vi "Set Temperature.vi"(8 "error in (no error)":errorcluster, 11 "CCDCamera in":refnum<class "CCDCamera.lvclass">) -> (0 "error out":errorcluster, 3 "CCDCamera out":refnum<class "CCDCamera.lvclass">)   [LabVIEW 2018, in "CCDCamera.lvclass"]
uses:
  CCDCamera.lvclass
  C:/Users/observer/Desktop/SPARC4_ACS/SPARC4_ACS/Simulated_CCD_Camera/Simulated_CCD_Camera.lvclass
  Simulated_CCD_Camera/Simulated_CCD_Camera.lvclass
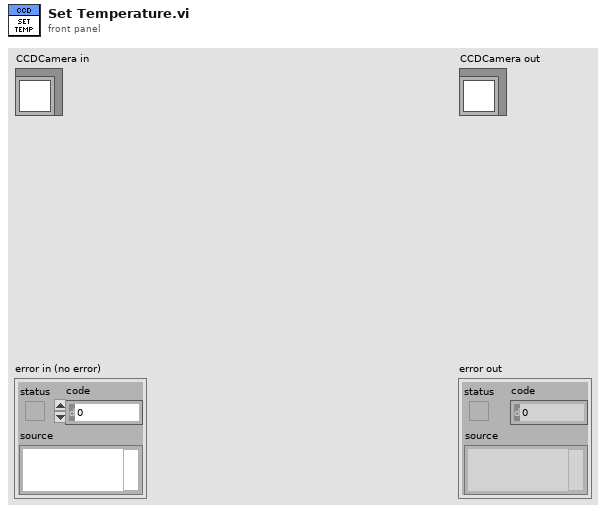
[diagram p1: front panel]
types:
  T1 = cluster{"COOLER_POWER_STATUS":u16, "TEMP":i32, "EXPTIME":sgl, "#FRAMES":u32, "#CUBES":u32}
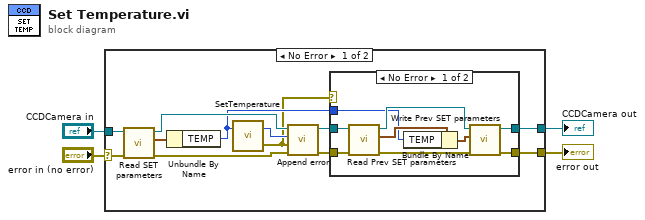
[diagram p0: block diagram]
diagram:
  n1 = case shown="No Error" "error in (no error)" {
    selector: "error in (no error)" -> [w16 w28]
    tunnel: "CCDCamera in" -> [w14 w29]
    tunnel: [w8 w29] -> w1
    tunnel: [w7 w28] -> w4
    frame No Error {
      n2 = call-dynamic "Read SET parameters.vi"("error in (no error)"=w16, "Simulated_CCD_Camera in"=w14) -> ("error out"=w12:errorcluster, "SET parameters"=w15:T1, "Simulated_CCD_Camera out"=w13:refnum<class "CCDCamera.lvclass">)  [unwired: 7 in]
      n3 = Unbundle By Name(w15) -> ("TEMP"=w6:i32)
      n4 = call <userlib>:"SetTemperature.vi"("temperature"=w6) -> ("error out"=w5:errorcluster, "DLL error code"=w11:u32)  [unwired: 1 in]
      n5 = call "Append error.vi"("error in (no error)"=w12, "error"=w5, "code"=w11, "Simulated_CCD_Camera in"=w13) -> ("error out"=w9:errorcluster, "Simulated_CCD_Camera out"=w10:refnum<class "CCDCamera.lvclass">)  [unwired: 6 in]
      n6 = case shown="No Error" w5 {
        tunnel: [w25 w27] -> w8
        tunnel: [w24 w26] -> w7
        tunnel: w10 -> [w20 w27]
        tunnel: w9 -> [w21 w26]
        tunnel: w6 -> [w17 _]
        frame No Error {
          n7 = call-dynamic "Read Prev SET parameters.vi"("error in (no error)"=w21, "Simulated_CCD_Camera in"=w20) -> ("error out"=w22:errorcluster, "Prev SET parameters"=w19:T1, "Simulated_CCD_Camera out"=w23:refnum<class "CCDCamera.lvclass">)  [unwired: 7 in]
          n8 = Bundle By Name(cluster=w19, "TEMP"=w17) -> (w18:T1)
          n9 = call-dynamic "Write Prev SET parameters.vi"("error in (no error)"=w22, "Prev SET parameters"=w18, "Simulated_CCD_Camera in"=w23) -> ("error out"=w24:errorcluster, "Simulated_CCD_Camera out"=w25:refnum<class "CCDCamera.lvclass">)  [unwired: 7 in]
        }
        frame Error {
        }
      }
    }
    frame Error {
    }
  }
  "error out" <- w4
  "CCDCamera out" <- w1
